vi "FTW-ActorExtended-Child-Get.vi"(0 "FTW-ActorExtended In":refnum<class "FTW-ActorExtended.lvclass">, 5 "Connector Name":string, 11 "error in":errorcluster) -> (4 "FTW-ActorExtended Out":refnum<class "FTW-ActorExtended.lvclass">, 6 "FTW Actor Connector":refnum<class "FTW-ActorConnector.lvclass">, 15 "error out":errorcluster)   [LabVIEW 2013, in "FTW-ActorExtended.lvclass"]
uses:
  FTW-ActorExtended.lvclass
  Connector/FTW-ActorConnector.lvclass
  FTW-ActorExtended.lvclass/FTW-ActorExtended.ctl
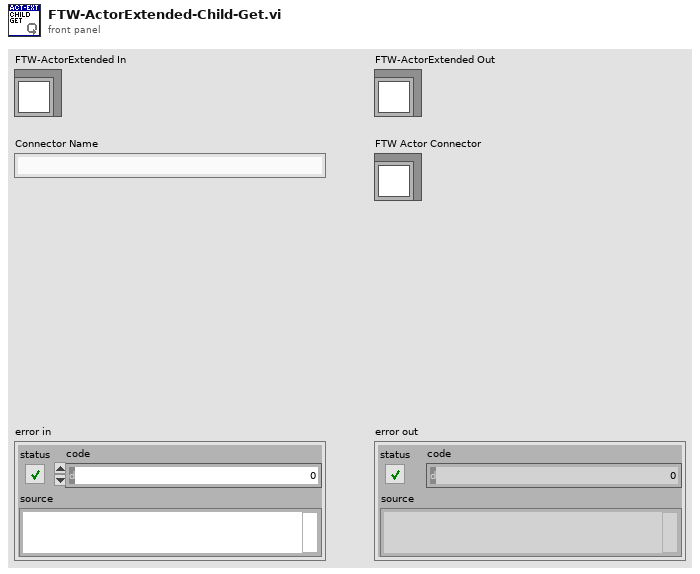
[diagram p1: front panel]
types:
  T1 = cluster{"Name":string, "URI":string, "Connector":refnum<class "FTW-ActorConnector.lvclass">, "Child":bool}[]
  T2 = cluster{"Name":string, "URI":string, "Connector":refnum<class "FTW-ActorConnector.lvclass">, "Child":bool}
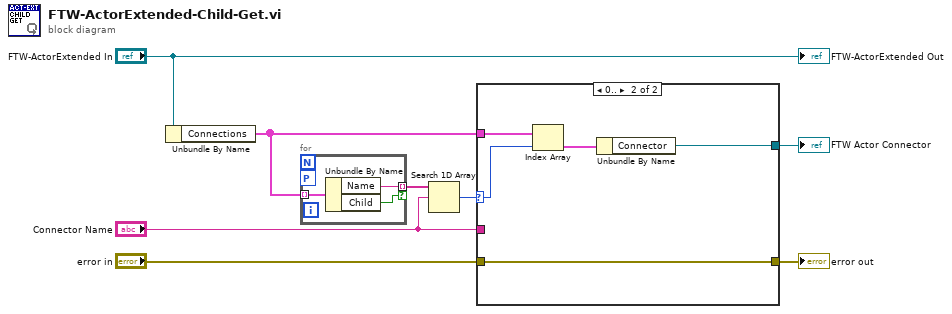
[diagram p0: block diagram]
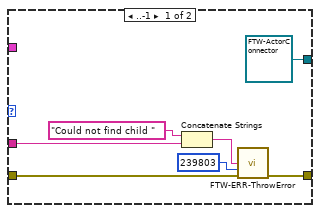
[diagram p2: hidden frame]
diagram:
  n1 = Unbundle By Name("FTW-ActorExtended In") -> ("Connections"=w6:T1)
  n2 = for {
    tunnel: w6 -> [w11] mode=indexing
    tunnel: [w10] -> w2 mode=indexing if=w9
    workers-P: _ -> [_]
    n3 = Unbundle By Name(w11) -> ("Name"=w10:string, "Child"=w9:bool)
  }
  n4 = Search 1D Array(1D array=w2, element="Connector Name") -> (index of element=w7:i32)  [unwired: 1 in]
  n5 = case shown="0.." w7 {
    selector: w7 -> [_ w23]
    tunnel: w6 -> [_ w22]
    tunnel: [w17 w21] -> w5
    tunnel: "error in" -> [w18 w21]
    tunnel: "Connector Name" -> [w13 _]
    tunnel: [refnum<class "FTW-ActorConnector.lvclass"> refnum ("Connector") w19] -> w1
    frame ..-1 {
      n6 = Concatenate Strings("Could not find child " ("Error Message"), w13) -> (w14:string)
      n7 = call "FTW-ERR-ThrowError.vi"("Error Message"=w14, "Error Code"=239803, "error in"=w18) -> ("error out"=w17:errorcluster)  [unwired: 12 in]
    }
    frame 0.. {
      n8 = Index Array(array=w22, index=w23) -> (element=w20:T2)
      n9 = Unbundle By Name(w20) -> ("Connector"=w19:refnum<class "FTW-ActorConnector.lvclass">)
    }
  }
  "error out" <- w5
  "FTW Actor Connector" <- w1
  "FTW-ActorExtended Out" <- "FTW-ActorExtended In"
